vi "Memory.Pointer.Write.Safe (1D U8).vi"(8 "error in (no error)":errorcluster, 9 "offset (0)":u64 format="%d bytes", 10 "buffer":u8[](array[numeric]) format="%02x", 11 "Pointer in":refnum<class "Memory.Pointer.lvclass">) -> (0 "error out":errorcluster, 1 "offset dup":u64 format="%d bytes", 2 "buffer dup":u8[](array[numeric]) format="%02x", 3 "Pointer out":refnum<class "Memory.Pointer.lvclass">)   [LabVIEW 2016, in "LabVIEW Memory Manager.lvlib" / "Memory.Pointer.lvclass"]
uses:
  Memory.Pointer.lvclass
  Memory.Pointer.Offset to Address.Safe.vi
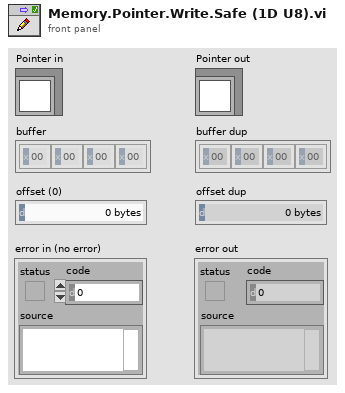
[diagram p1: front panel]
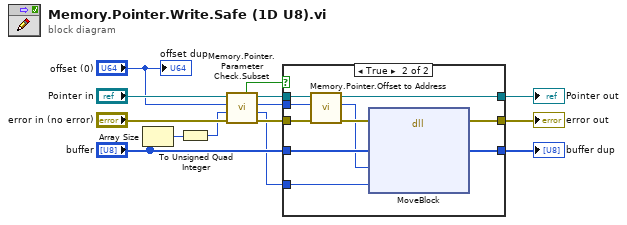
[diagram p0: block diagram]
diagram:
  n1 = Array Size(array="buffer") -> (size(s)=w12:i32)
  n2 = To Unsigned Quad Integer(1:w12) -> (0:w3:u64)
  n3 = call "Memory.Pointer.Parameter Check.Subset.vi"("error in (no error)"="error in (no error)", "length"=w3, "offset"="offset (0)", "Pointer in"="Pointer in") -> ("error out"=w5:errorcluster, "length out"=w2:u64, "offset out"=w4:u64, "Pointer out"=w6:refnum<class "Memory.Pointer.lvclass">, "subset valid"=w1:bool)  [unwired: 3 in]
  n4 = case shown="True" w1 {
    tunnel: [w17 w27] -> w14
    tunnel: [w16 w26] -> w13
    tunnel: [w15 w24] -> w11
    tunnel: "buffer" -> [w15 w19]
    tunnel: w6 -> [w17 w23]
    tunnel: w5 -> [w16 w22]
    tunnel: w4 -> [_ w21]
    tunnel: w2 -> [_ w20]
    frame False {
    }
    frame True {
      n5 = call-poly "Memory.Pointer.Offset to Address.vi"("error in (no error)"=w22, "offset"=w21, "Pointer in"=w23) -> ("error out"=w25:errorcluster, "address"=w18:u64, "Pointer out"=w27:refnum<class "Memory.Pointer.lvclass">)  [unwired: 6 in]
      n6 = dll-call lib="LabVIEW" fn="MoveBlock"(error in=w25, "src pointer"=w19, "dst pointer"=w18, "size"=w20) -> (error out=w26:errorcluster, "src pointer"=w24:u8[])  [unwired: 5 in, 1 out]
    }
  }
  "error out" <- w13
  "Pointer out" <- w14
  "buffer dup" <- w11
  "offset dup" <- "offset (0)"
